vi "FT10_Unitherm Open Connection.vi"(8 "error in (no error)":errorcluster, 11 "VISA Refnum in":refnum<visa-resource-name>="COM4") -> (0 "error out":errorcluster, 3 "VISA Refnum out":refnum<visa-resource-name>="COM4")   [LabVIEW 2015]
uses:
  <vilib>/Instr/_visa.llb/VISA Configure Serial Port (Instr).vi
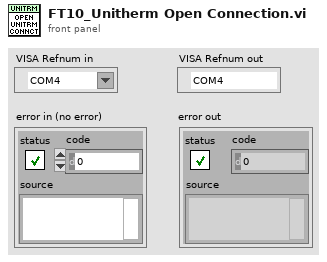
[diagram p1: front panel]
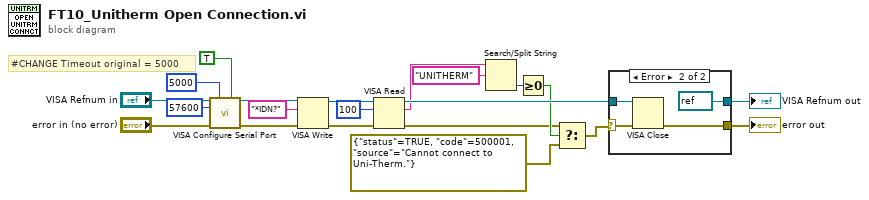
[diagram p0: block diagram]
diagram:
  # "#CHANGE Timeout original = 5000"
  n1 = call-poly "VISA Configure Serial Port"("VISA resource name"="VISA Refnum in", "timeout (10sec)"=u32 5000, "Enable Termination\nChar (T)"=TRUE ("Enable Termination\nChar (T)"), "baud rate (9600)"=u32 57600, "error in (no error)"="error in (no error)") -> ("VISA resource name out"=w11:refnum<visa-resource-name>, "error out"=w10:errorcluster)  [unwired: 9 in]
  n2 = VISA Write(VISA resource name=w11, write buffer="*IDN?" ("string"), error in (no error)=w10) -> (VISA resource name out=w15:refnum<visa-resource-name>, error out=w14:errorcluster)  [unwired: 1 out]
  n3 = VISA Read(VISA resource name=w15, byte count=u32 100, error in (no error)=w14) -> (VISA resource name out=w18:refnum<visa-resource-name>, read buffer=w6:string, error out=w1:errorcluster)  [unwired: 1 out]
  n4 = Search/Split String(string=w6, search string/char (-)="UNITHERM") -> (offset of match=w4:i32)  [unwired: 1 in, 2 out]
  n5 = Greater Or Equal To 0?(x=w4) -> (x >= 0?=w3:bool)
  n6 = Select(t=w1, s=w3, f=errorcluster {"status"=TRUE, "code"=500001, "source"="Cannot connect to Uni-Therm."} ("error constant")) -> (s? t:f=w17:errorcluster)
  n7 = case shown="Error" w17 {
    selector: w17 -> [w22 w26]
    tunnel: w18 -> [w23 w24]
    tunnel: [w23 refnum<visa-resource-name> refnum ("VISA resource name out")] -> w20
    tunnel: [w22 w25] -> w19
    frame No Error {
    }
    frame Error {
      n8 = VISA Close(VISA resource name=w24, error in (no error)=w26) -> (error out=w25:errorcluster)
    }
  }
  "error out" <- w19
  "VISA Refnum out" <- w20
